vi "API.vi"() -> ()   [LabVIEW 2018]
uses:
  dd124b5f-36c7-4e7c-bcc8-37bfffb7cae4.vi
  8ea95075-ec7b-4070-b8fa-2f3b772012e4.vi
  c5faf44e-6c66-4be6-bc49-170f88b0dffb.vi
  72defa96-1dad-4704-b983-8c3a2842dd53.vi
  62821ff5-7b51-4fb3-8449-2ccbb7cfd9cf.vi
  a345b58e-fa81-498b-941c-1bfe72ced7b2.vi
  27b3211a-0c0d-41bc-ab24-ed8bc60d9a3e.vi
  6ff51e3a-8f52-4f4b-8c43-8d4f807ed1ff.vi
  9bf46c02-7a8f-4e83-8ee1-f8cedbfdb624.vi
  6536fed6-d68e-4967-8e6a-e2def0745587.vi
  6fa4e6d2-d40c-4a7c-8a57-a21af05c07b8.vi
  d3567d77-016b-4747-ae39-8267dda81e1a.vi
  e2d3a09e-3eda-43e4-847b-f5ba23d2d1dd.vi
  b105d130-1003-4e1c-a69e-171ed3b4cd62.vi
  7eaf2191-3900-4e37-b8f1-0b56292f964b.vi
  164712d4-a40f-4c1d-9dd6-f0e909c7f9ac.vi
  f83999bd-597e-49a3-8a24-f514c2e803fa.vi
  ef0be5a8-4980-411d-972c-ca998a3188ce.vi
  dd124b5f-36c7-4e7c-bcc8-37bfffb7cae4.vi/5ce1af88-85f0-419a-8d80-1694d27860f0.vi
  8ea95075-ec7b-4070-b8fa-2f3b772012e4.vi/5a01e313-fc7d-4519-ba39-81d8e4580f6b.vi
  c5faf44e-6c66-4be6-bc49-170f88b0dffb.vi/a06e9705-c341-4fd3-ab56-b0df9b5f3d25.vi
  72defa96-1dad-4704-b983-8c3a2842dd53.vi/a153a250-4fb8-4a99-bb5b-6ccb57f1f631.vi
  62821ff5-7b51-4fb3-8449-2ccbb7cfd9cf.vi/a02c6254-97f5-44e3-a3a9-7fdb6dfbd055.vi
  a345b58e-fa81-498b-941c-1bfe72ced7b2.vi/bae24b8d-f663-491e-8374-2218e527d0d0.vi
  27b3211a-0c0d-41bc-ab24-ed8bc60d9a3e.vi/083db1d9-8cf1-45e4-a540-e8e178cc7cc8.vi
  6ff51e3a-8f52-4f4b-8c43-8d4f807ed1ff.vi/083db1d9-8cf1-45e4-a540-e8e178cc7cc8.vi
  9bf46c02-7a8f-4e83-8ee1-f8cedbfdb624.vi/083db1d9-8cf1-45e4-a540-e8e178cc7cc8.vi
  6536fed6-d68e-4967-8e6a-e2def0745587.vi/bf655d3c-1ce4-400f-a78f-0f3f0191886e.vi
  Mark Error.vi
  6fa4e6d2-d40c-4a7c-8a57-a21af05c07b8.vi/de1063af-56d8-4a46-86b0-d7db6137800f.vi
  d3567d77-016b-4747-ae39-8267dda81e1a.vi/ba94d47b-0e30-4c32-b8ff-86d609cd95a5.vi
  b105d130-1003-4e1c-a69e-171ed3b4cd62.vi/7453dcce-b283-4a0d-ab92-51c518b086c4.vi
  7eaf2191-3900-4e37-b8f1-0b56292f964b.vi/083db1d9-8cf1-45e4-a540-e8e178cc7cc8.vi
  164712d4-a40f-4c1d-9dd6-f0e909c7f9ac.vi/28727e37-b0d9-407c-a479-ab0b7779cd69.vi
  72defa96-1dad-4704-b983-8c3a2842dd53.vi/a153a250-4fb8-4a99-bb5b-6ccb57f1f631.vi/28727e37-b0d9-407c-a479-ab0b7779cd69.vi
  62821ff5-7b51-4fb3-8449-2ccbb7cfd9cf.vi/a02c6254-97f5-44e3-a3a9-7fdb6dfbd055.vi/7453dcce-b283-4a0d-ab92-51c518b086c4.vi
  a345b58e-fa81-498b-941c-1bfe72ced7b2.vi/bae24b8d-f663-491e-8374-2218e527d0d0.vi/083db1d9-8cf1-45e4-a540-e8e178cc7cc8.vi
  Registry/Log.vi
  0dfa3e82-4891-44d4-bf0f-fa00f786f96a.vi
  bb7e9841-758c-4434-a6dd-f489ab997295.vi
  83cdd324-15c3-40f2-bb86-434760b938a2.vi
  3f72ac97-b943-4619-9f88-611e59474e32.vi
panel:
  out "double out":dbl format="%.2f"
  out "integer out":i32
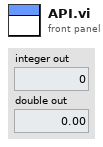
[diagram p1: front panel]
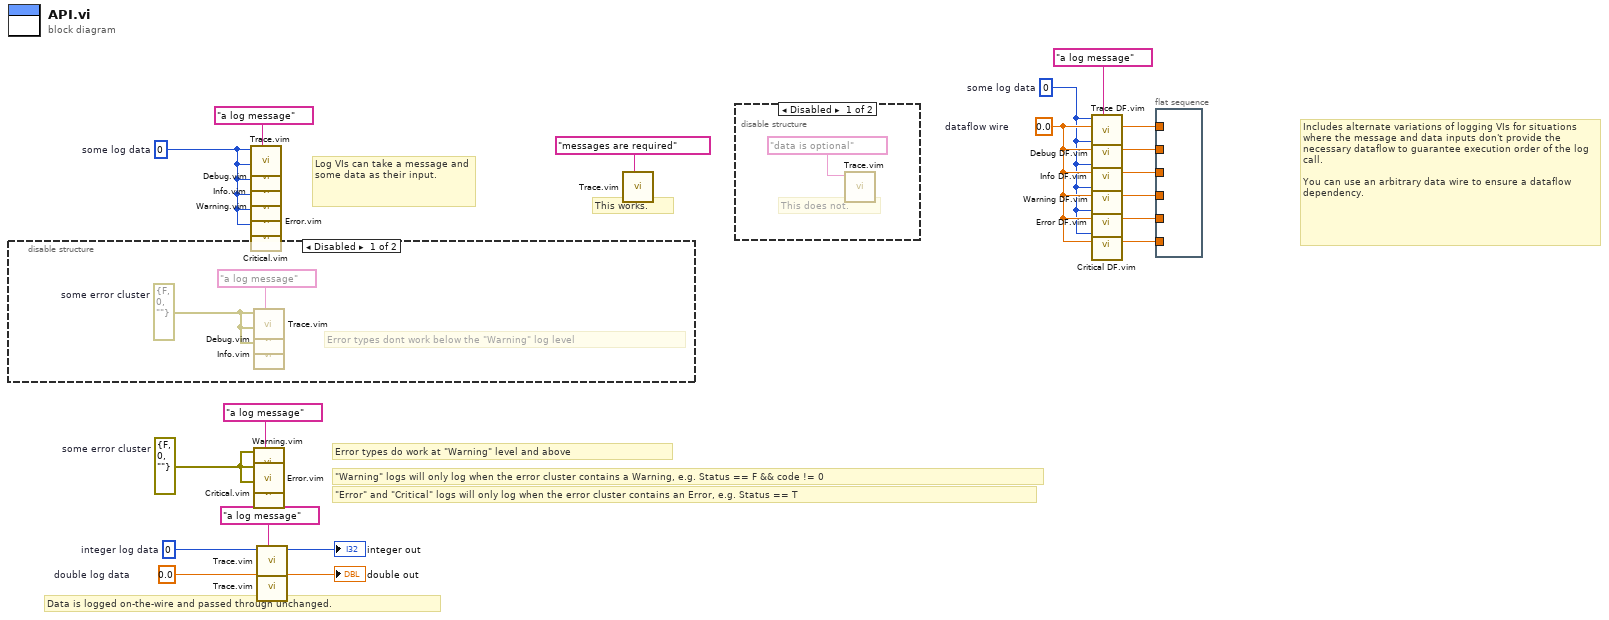
[diagram p0: block diagram]
diagram:
  w8 = 0.0  # dataflow wire
  w11 = "a log message"
  w3 = 0  # some log data
  w14 = 0.0  # double log data
  w17 = 0  # integer log data
  w13 = "a log message"
  w1 = "a log message"
  w2 = errorcluster {"status"=FALSE, "code"=0, "source"=""}  # some error cluster
  w18 = 0  # some log data
  w19 = "a log message"
  # "\"Error\" and \"Critical\" logs will only log when the error cluster contains an Error, e.g. Status == T"
  # "\"Warning\" logs will only log when the error cluster contains a Warning, e.g. Status == F && code != 0"
  # "Includes alternate variations of logging VIs for situations where the message and data inputs don't provide the necessary dataflow to guarantee execution order of the log call.\n\nYou can use an arbitrary data wire to ensure a dataflow dependency."
  # "This works."
  # "Log VIs can take a message and some data as their input."
  # "Data is logged on-the-wire and passed through unchanged."
  # "Error types do work at \"Warning\" level and above"
  n1 = disable-structure shown="Disabled" {
    frame Disabled {
      w20 = errorcluster {"status"=FALSE, "code"=0, "source"=""}  # some error cluster
      w21 = "a log message"
      # "Error types dont work below the \"Warning\" log level"
      n2 = call "Trace.vim"("data in (null)"=w20, "message"=w21) -> ()  [unwired: 9 in, 1 out]
      n3 = call "Debug.vim"("data in (null)"=w20, "message"=w21) -> ()  [unwired: 9 in, 1 out]
      n4 = call "Info.vim"("data in (null)"=w20, "message"=w21) -> ()  [unwired: 9 in, 1 out]
    }
    frame Enabled {
    }
  }
  n5 = call "Trace.vim"("data in (null)"=w18, "message"=w19) -> ()  [unwired: 9 in, 1 out]
  n6 = call "Debug.vim"("data in (null)"=w18, "message"=w19) -> ()  [unwired: 9 in, 1 out]
  n7 = call "Info.vim"("data in (null)"=w18, "message"=w19) -> ()  [unwired: 9 in, 1 out]
  n8 = call "Warning.vim"("data in (null)"=w18, "message"=w19) -> ()  [unwired: 9 in, 1 out]
  n9 = call "Error.vim"("data in (null)"=w18, "message"=w19) -> ()  [unwired: 9 in, 1 out]
  n10 = call "Critical.vim"("data in (null)"=w18, "message"=w19) -> ()  [unwired: 9 in, 1 out]
  n11 = call "Warning.vim"("data in (null)"=w2, "message"=w1) -> ()  [unwired: 9 in, 1 out]
  n12 = call "Error.vim"("data in (null)"=w2, "message"=w1) -> ()  [unwired: 9 in, 1 out]
  n13 = call "Critical.vim"("data in (null)"=w2, "message"=w1) -> ()  [unwired: 9 in, 1 out]
  n14 = call "Trace.vim"("data in (null)"=w17, "message"=w13) -> ("data out"=→"integer out":i32)  [unwired: 9 in]
  n15 = call "Trace.vim"("data in (null)"=w14, "message"=w13) -> ("data out"=→"double out":dbl)  [unwired: 9 in]
  n16 = call "Trace.vim"("message"="messages are required") -> ()  [unwired: 10 in, 1 out]
  n17 = disable-structure shown="Disabled" {
    frame Disabled {
      # "This does not."
      n18 = call "Trace.vim"("data in (null)"="data is optional") -> ()  [unwired: 10 in, 1 out]
    }
    frame Enabled {
    }
  }
  n19 = call "Trace DF.vim"("message"=w11, "dataflow in"=w8, "data (null)"=w3) -> ("dataflow out"=w10:dbl)  [unwired: 8 in]
  n20 = call "Debug DF.vim"("message"=w11, "dataflow in"=w8, "data (null)"=w3) -> ("dataflow out"=w9:dbl)  [unwired: 8 in]
  n21 = call "Info DF.vim"("message"=w11, "dataflow in"=w8, "data (null)"=w3) -> ("dataflow out"=w7:dbl)  [unwired: 8 in]
  n22 = call "Warning DF.vim"("message"=w11, "dataflow in"=w8, "data (null)"=w3) -> ("dataflow out"=w6:dbl)  [unwired: 8 in]
  n23 = call "Error DF.vim"("message"=w11, "dataflow in"=w8, "data (null)"=w3) -> ("dataflow out"=w5:dbl)  [unwired: 8 in]
  n24 = call "Critical DF.vim"("message"=w11, "dataflow in"=w8, "data (null)"=w3) -> ("dataflow out"=w4:dbl)  [unwired: 8 in]
  n25 = flat-sequence {
    tunnel: w10 -> [_]
    tunnel: w9 -> [_]
    tunnel: w7 -> [_]
    tunnel: w6 -> [_]
    tunnel: w5 -> [_]
    tunnel: w4 -> [_]
    frame #0 {
    }
  }
